vi "Finalize.vi"(8 "error in":errorcluster, 11 "Ballard ARINC-429 shared resources in":refnum<class "Shared Resources.lvclass">) -> (0 "error out":errorcluster, 3 "Ballard ARINC-429 shared resources out":refnum<class "Shared Resources.lvclass">)   [LabVIEW 2020, in "Ballard ARINC 429 Engine.lvlib" / "Implementation.lvlib" / "Shared Resources.lvclass"]
uses:
  Shared Resources.lvclass
  Custom Device/Custom Device.lvlib
  Custom Device/Hardware Handles.ctl
  Logging/Word Logging/Word Logging.lvlib
  Logging/Word Logging/Log Producer/Log Producer.lvclass
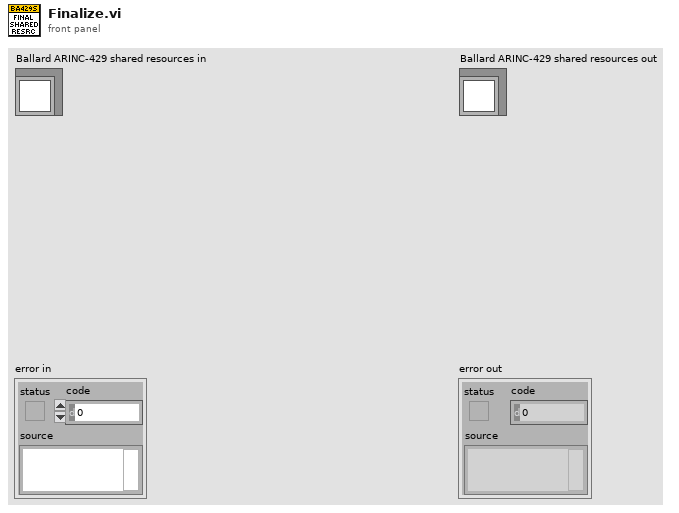
[diagram p1: front panel]
types:
  T1 = typedef "Ballard ARINC 429 Engine.lvlib/Custom Device.lvlib/Hardware Handles.ctl" = cluster{"core handle":u64, "core reader handle":u64, "channel handles":u64[]}
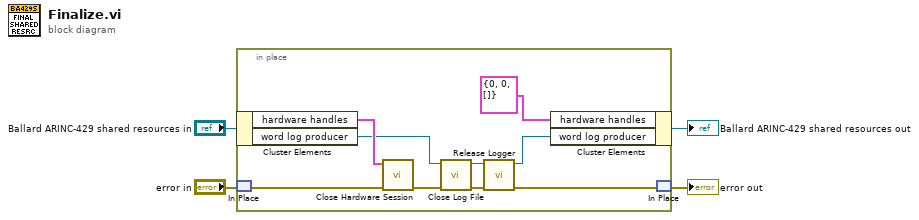
[diagram p0: block diagram]
diagram:
  n1 = in-place {
    n2 = in-place-cluster #1("Ballard ARINC-429 shared resources in") -> ("hardware handles"=w13:T1, "word log producer"=w6:refnum<class "Log Producer.lvclass">)
    n3 = in-place-match #2("error in") -> (w12:errorcluster)
    n4 = call "Close Hardware Session.vi"("error in"=w12, "hardware handles"=w13) -> ("error out"=w11:errorcluster)  [unwired: 9 in]
    n5 = call "Close Log File.vi"("error in (no error)"=w11, "Log Producer in"=w6) -> ("error out"=w7:errorcluster, "Log Producer out"=w5:refnum<class "Log Producer.lvclass">)  [unwired: 8 in]
    n6 = call "Release Logger.vi"("error in (no error)"=w7, "Producer"=w5) -> ("error out"=w9:errorcluster, "Default Producer"=w8:refnum<class "Log Producer.lvclass">)  [unwired: 8 in]
    n7 = in-place-cluster #1("hardware handles"=T1 {"core handle"=0, "core reader handle"=0, "channel handles"=[]} ("RT handles"), "word log producer"=w8) -> (→"Ballard ARINC-429 shared resources out":refnum<class "Shared Resources.lvclass">)
    n8 = in-place-match #2(w9) -> (→"error out":errorcluster)
  }
